vi "4.6.2.vi"() -> ()   [LabVIEW 2017]
panel:
  in  "停止":bool
  in  "x":dbl
  out "结果":dbl
  in  "y":dbl
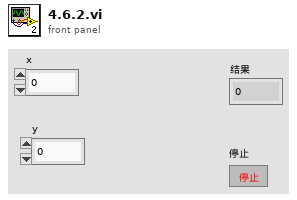
[diagram p1: front panel]
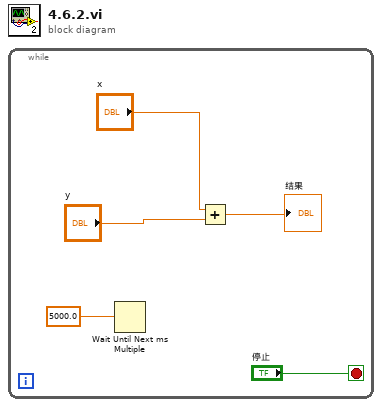
[diagram p0: block diagram]
diagram:
  n1 = while {
    stop <- "停止" stop-if-true
    n2 = Wait Until Next ms Multiple(millisecond multiple=5000.0) -> ()  [unwired: 1 out]
    n3 = Add(x="x", y="y") -> (x+y=→"结果":dbl)
  }
